vi "MongoDB.FindOneSorted.vi"(8 "error in (no error)":errorcluster, 10 "Sort Keys":string[](array[string])=["_id"], 11 "MongoDB.Collection in":refnum<class "MongoDB.Collection.lvclass">) -> (0 "error out":errorcluster, 2 "Result":string, 3 "MongoDB.Collection out":refnum<class "MongoDB.Collection.lvclass">)   [LabVIEW 2014, in "MongoDB.Collection.lvclass"]
uses:
  MongoDB.Collection.lvclass
  C:/Users/Richard/Documents/GitHub/mongo-labview-driver/CSharp/bin/MongoDB.Driver.Legacy.dll
  CSharp/bin/MongoDB.Driver.Legacy.dll
  MongoDB.Collection.lvclass/MongoDB.Collection.ctl
  C:/Users/Richard/Documents/GitHub/mongo-labview-driver/CSharp/bin/MongoDB.Bson.dll
  CSharp/bin/MongoDB.Bson.dll
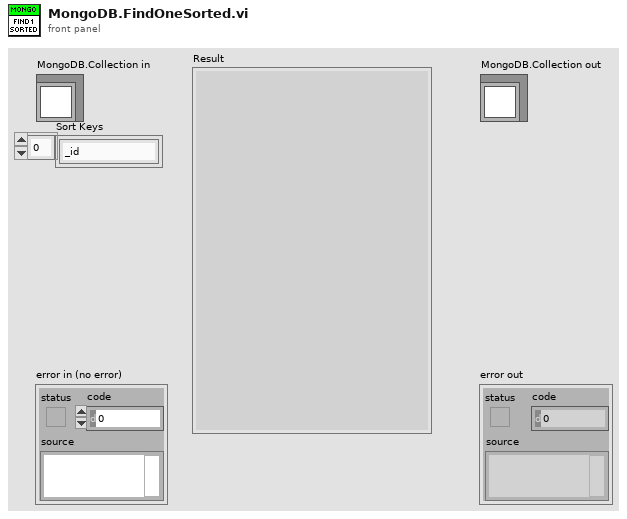
[diagram p1: front panel]
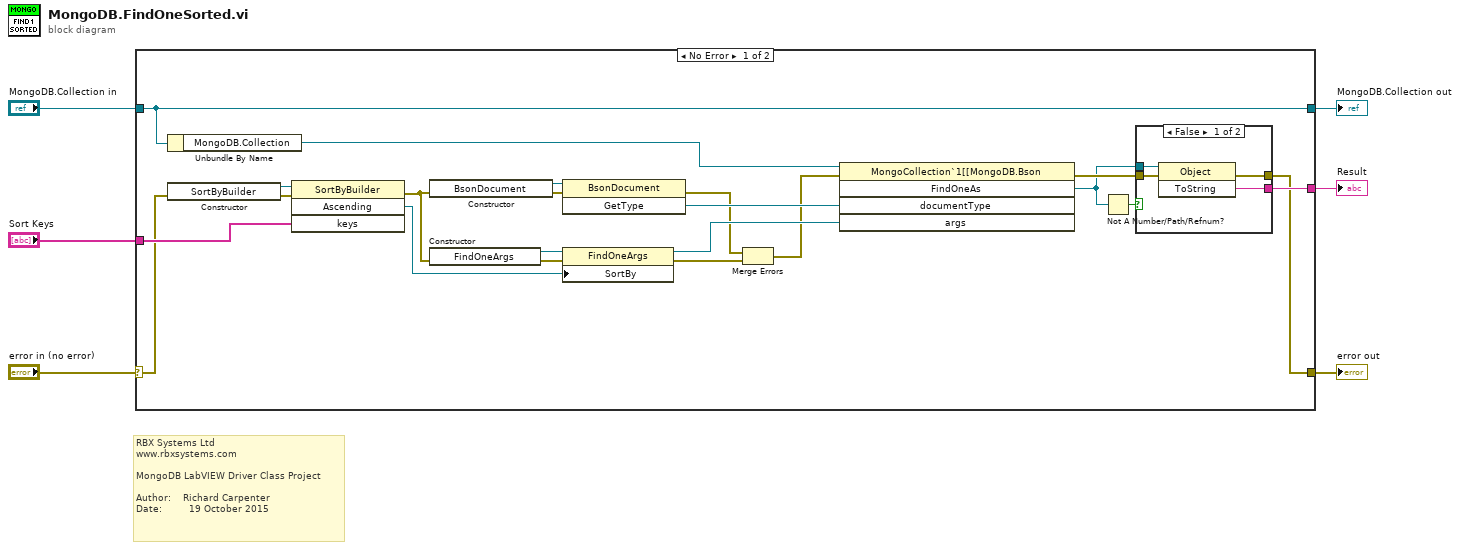
[diagram p0: block diagram]
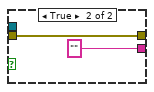
[diagram p2: hidden frame]
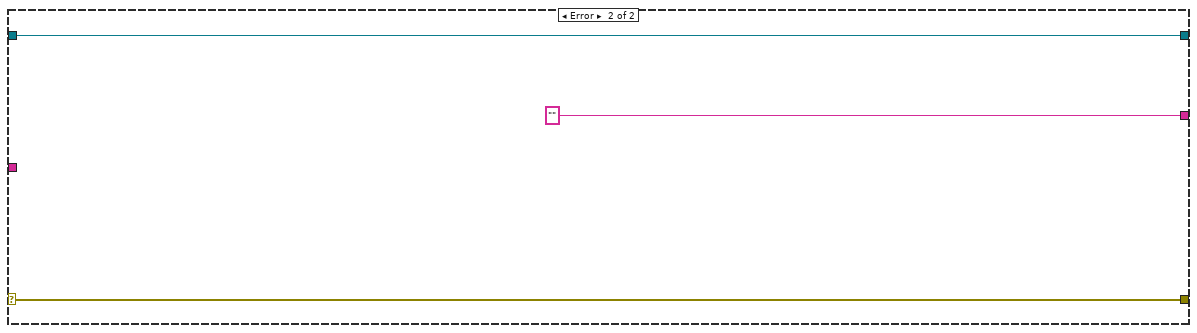
[diagram p3: hidden frame]
diagram:
  # "RBX Systems Ltd\nwww.rbxsystems.com\n\nMongoDB LabVIEW Driver Class Project\n\nAuthor:    Richard Carpenter\nDate:         19 October 2015"
  n1 = case shown="No Error" "error in (no error)" {
    selector: "error in (no error)" -> [w13 w37]
    tunnel: [w26 w37] -> w5
    tunnel: [w28 w36] -> w3
    tunnel: "MongoDB.Collection in" -> [w28 w36]
    tunnel: [w27 "" ("AsString")] -> w2
    tunnel: "Sort Keys" -> [w14 _]
    frame No Error {
      n2 = Unbundle By Name(w28) -> ("MongoDB.Collection"=w18:refnum<k24>)
      n3 = constructor class="SortByBuilder"(error in=w13) -> (reference out=w24:refnum<k24>, error out=w15:errorcluster)  [unwired: 2 in, 1 out]
      n4 = invoke class="SortByBuilder" method="Ascending"(reference=w24, error in=w15, "keys"=w14) -> (error out=w10:errorcluster, "Ascending"=w22:refnum<k24>)  [unwired: 1 in, 2 out]
      n5 = constructor class="BsonDocument"(error in=w10) -> (reference out=w20:refnum<k24>, error out=w12:errorcluster)  [unwired: 2 in, 1 out]
      n6 = constructor class="FindOneArgs"(error in=w10) -> (reference out=w23:refnum<k24>, error out=w11:errorcluster)  [unwired: 2 in, 1 out]
      n7 = invoke class="BsonDocument" method="GetType"(reference=w20, error in=w12) -> (error out=w9:errorcluster, "GetType"=w19:refnum<k24>)  [unwired: 1 in, 1 out]
      n8 = property class="FindOneArgs"(reference=w23, error in=w11, "SortBy"=w22) -> (reference out=w21:refnum<k24>, error out=w8:errorcluster)
      n9 = Merge Errors(w9, w8) -> (w7:errorcluster)
      n10 = invoke class="MongoCollection`1[[MongoDB.Bson" method="FindOneAs"(reference=w18, error in=w7, "documentType"=w19, "args"=w21) -> (error out=w17:errorcluster, "FindOneAs"=w16:refnum<k24>)  [unwired: 1 in, 3 out]
      n11 = Not A Number/Path/Refnum?(number/path/refnum=w16) -> (NaN/Path/Refnum?=w25:bool)
      n12 = case shown="False" w25 {
        tunnel: [w29 "" ("AsString")] -> w27
        tunnel: w16 -> [w32 _]
        tunnel: w17 -> [w31 w33]
        tunnel: [w30 w33] -> w26
        frame False {
          n13 = invoke class="Object" method="ToString"(reference=w32, error in=w31) -> (error out=w30:errorcluster, "ToString"=w29:string)  [unwired: 1 in, 1 out]
        }
        frame True {
        }
      }
    }
    frame Error {
    }
  }
  "error out" <- w5
  "MongoDB.Collection out" <- w3
  "Result" <- w2
